vi "Abrir PDF dentro de labview.vi"(0 "PDF file":path, 5 "error in (no error)":errorcluster) -> (19 "error out":errorcluster)   [LabVIEW 2019]
doc: "Use this VI to display a PDF document in a dialog box.\nIn the <B>PDF file</B> text box, enter the path to the PDF you want to display, or click the <B>Browse</B> button to navigate to a file.\nClick the <B>Run</B> button to view the PDF in the <B>PDF display</B>.\nClick the <B>Stop</B> button to stop the VI and remove the PDF from display."
panel:
  in  "STOP":bool
  in  "AcroPDF":refnum<k7>(container)
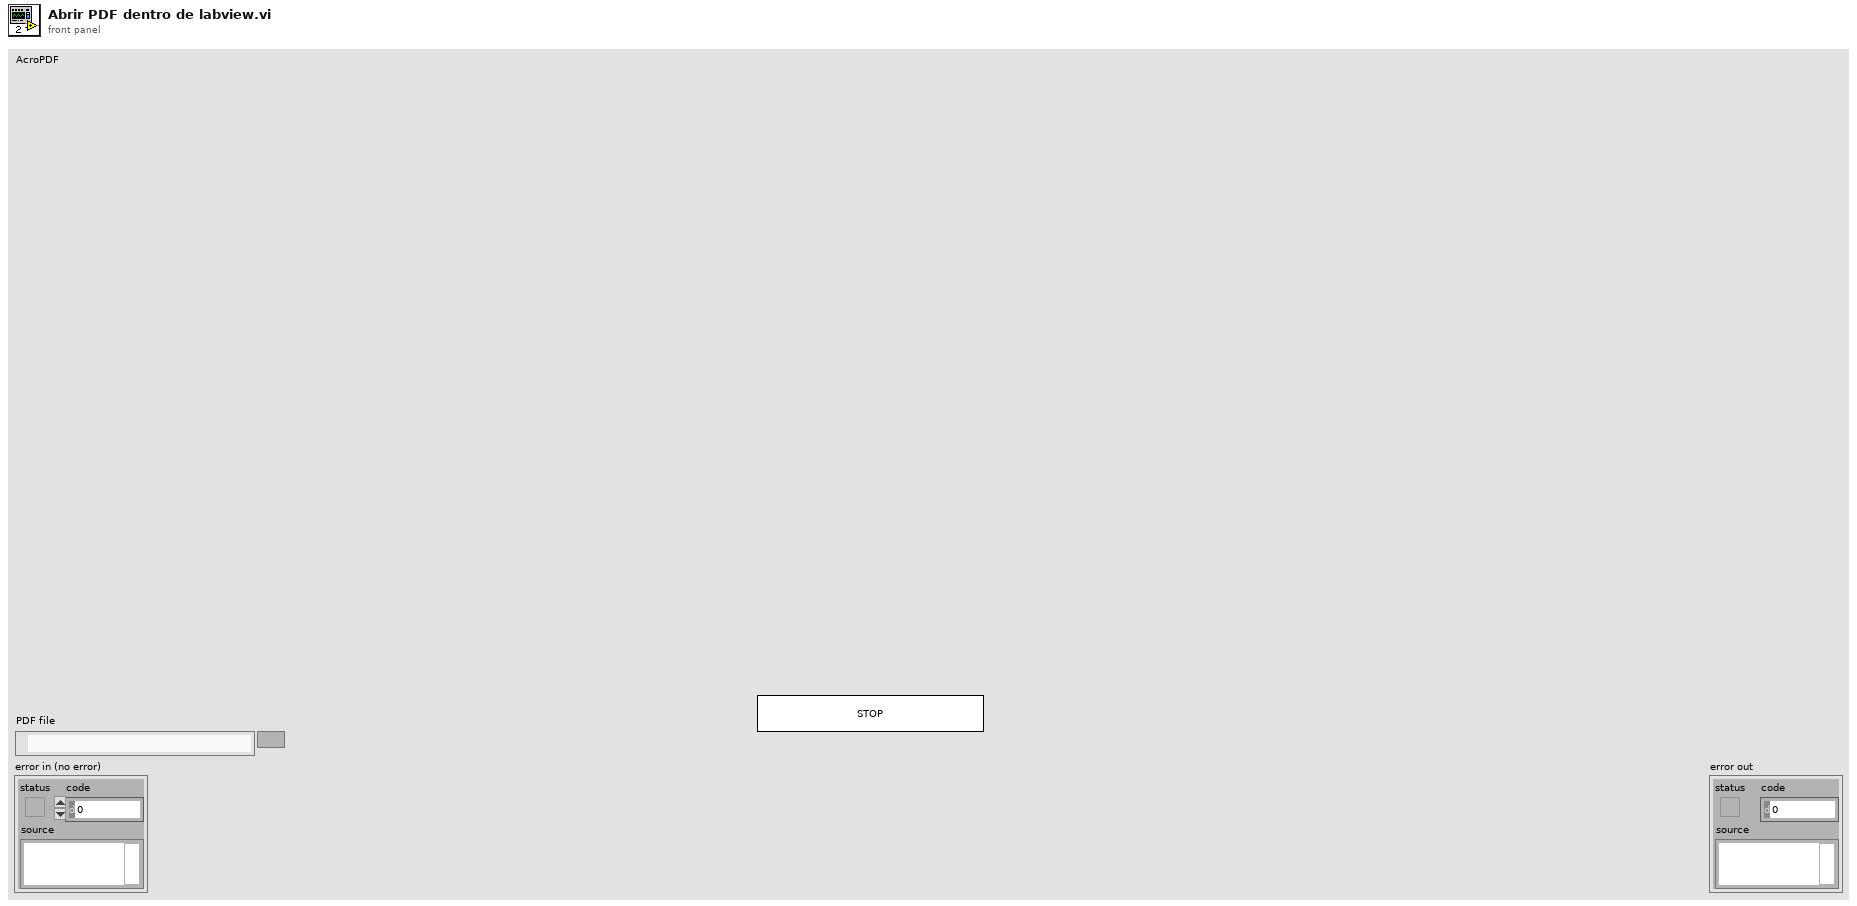
[diagram p1: front panel]
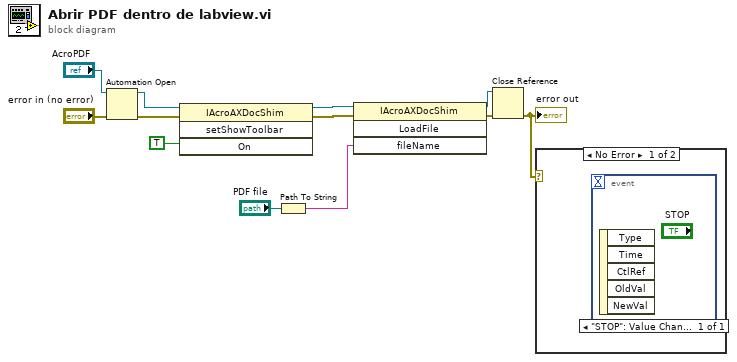
[diagram p0: block diagram]
diagram:
  n1 = Automation Open(error in (no error)="error in (no error)", Automation Refnum="AcroPDF") -> (Automation Refnum=w3:refnum<k7>, error out=w1:errorcluster)  [unwired: 2 in]
  n2 = invoke class="IAcroAXDocShim" method="setShowToolbar"(reference=w3, error in=w1, "On"=TRUE) -> (reference out=w6:refnum<k7>, error out=w5:errorcluster)  [unwired: 1 in, 2 out]
  n3 = Path To String(path="PDF file") -> (string=w10:string)
  n4 = invoke class="IAcroAXDocShim" method="LoadFile"(reference=w6, error in=w5, "fileName"=w10) -> (reference out=w12:refnum<k7>, error out=w11:errorcluster)  [unwired: 1 in, 2 out]
  n5 = Close Reference(reference=w12, error in (no error)=w11) -> (error out=w8:errorcluster)
  "error out" <- w8
  n6 = case shown="No Error" w8 {
    frame No Error {
      n7 = event shown="[0] \"STOP\": Value Change" {
        selector: _ -> [_]
        dyn-events: _ -> [_]
        timeout: _ -> [_]
        event "STOP": Value Change {
          n8 = event-data() -> ()  [unwired: 1 in, 5 out]
        }
      }
    }
    frame Error {
    }
  }
